vi "Boolean Case Structure.vi"() -> ()   [LabVIEW 2023]
panel:
  in  "Fahrenheit?":bool
  in  "stop":bool
  out "Temperature Output":dbl(slide) scale=0.0..2000.0
  in  "Celsius Input":dbl(slide) scale=0.0..1000.0
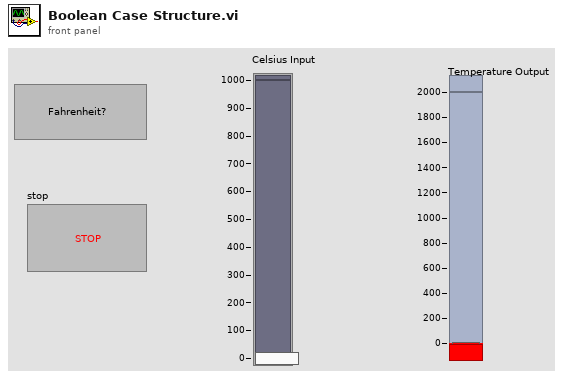
[diagram p1: front panel]
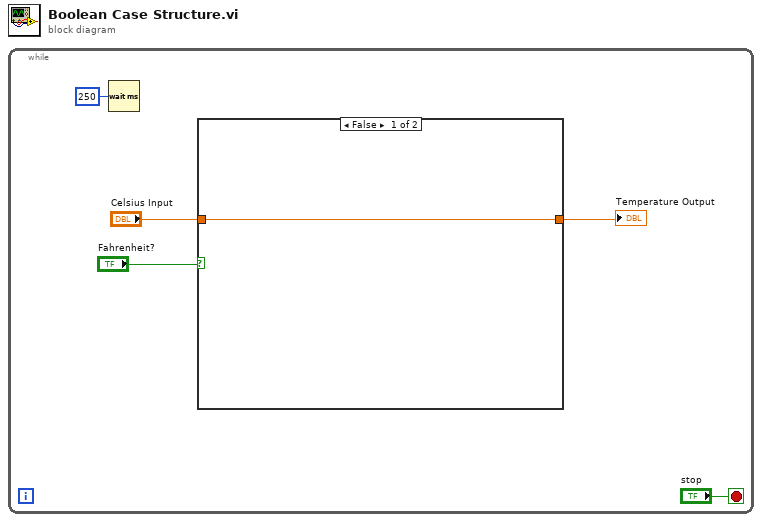
[diagram p0: block diagram]
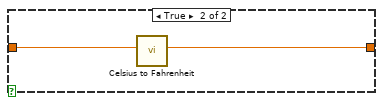
[diagram p2: hidden frame]
diagram:
  n1 = while {
    stop <- "stop" stop-if-true
    n2 = Wait (ms)(milliseconds to wait=u32 250) -> ()  [unwired: 1 out]
    n3 = case shown="False" "Fahrenheit?" {
      tunnel: "Celsius Input" -> [w6 w8]
      tunnel: [w6 w7] -> w2
      frame False {
      }
      frame True {
        n4 = call "Celsius to Fahrenheit.vi"("Celsius"=w8) -> ("Fahrenheit"=w7:dbl)  [unwired: 10 in]
      }
    }
    "Temperature Output" <- w2
  }
